vi "DiffDrivePoseEst2_Trajectory_SetAuto.vi"(11 "Ramsete AUTO":bool) -> ()   [LabVIEW 2019]
uses:
  DiffDrivePoseEst2_Trajectory_Globals.vi
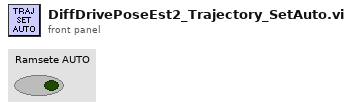
[diagram p1: front panel]
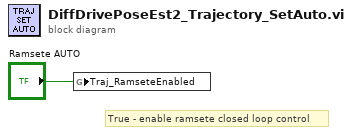
[diagram p0: block diagram]
diagram:
  # "True - enable ramsete closed loop control"
  n1 = global write "DiffDrivePoseEst2_Trajectory_Globals.vi" "Traj_RamseteEnabled"("Ramsete AUTO") -> ()
